vi "Manual Calibration.vi"(6 "Fresh Fill Density (V)":dbl, 9 "Brine Fill Density (V)":dbl, 10 "Fresh Density (kg/m3) 3":dbl, 11 "Brine Density (kg/m3)":dbl) -> (2 "Numeric 2":dbl, 3 "Numeric":dbl)   [LabVIEW 2011]
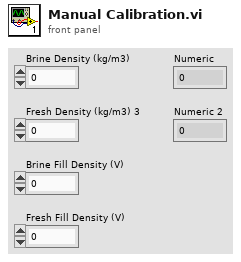
[diagram p1: front panel]
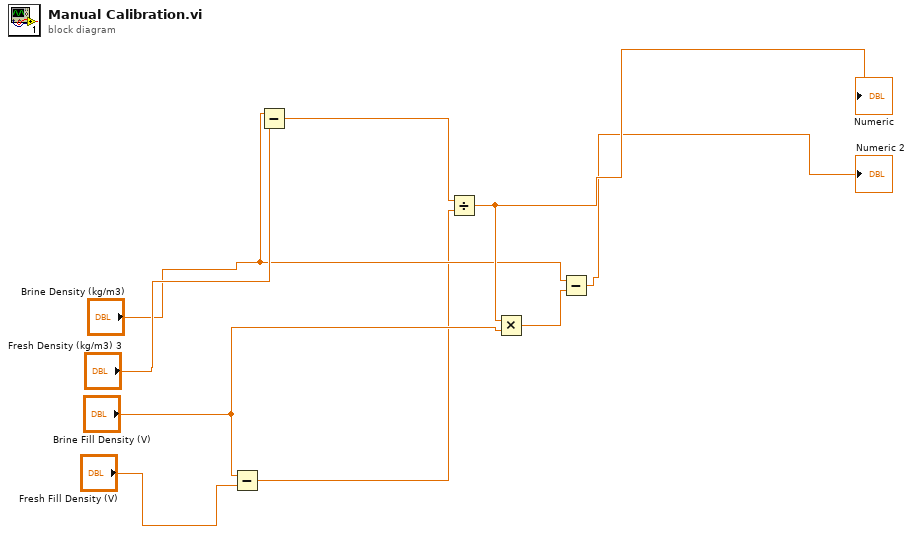
[diagram p0: block diagram]
diagram:
  n1 = Subtract(x="Brine Fill Density (V)", y="Fresh Fill Density (V)") -> (x-y=w1:dbl)
  n2 = Subtract(x="Brine Density (kg/m3)", y="Fresh Density (kg/m3) 3") -> (x-y=w2:dbl)
  n3 = Divide(x=w2, y=w1) -> (x/y=w9:dbl)
  "Numeric" <- w9
  n4 = Multiply(x=w9, y="Brine Fill Density (V)") -> (x*y=w3:dbl)
  n5 = Subtract(x="Brine Density (kg/m3)", y=w3) -> (x-y=→"Numeric 2":dbl)
